vi "2D_rotate.vi"(8 "error in (no error)":errorcluster, 10 "angle":dbl[unit], 11 "input vector":dbl[](array[numeric])) -> (0 "error out":errorcluster, 3 "output vector":dbl[](array[numeric]))   [LabVIEW 2010]
uses:
  <vilib>/Analysis/Matrix/Numeric/Conversions/Array To Matrix - RA2.vi
  <vilib>/Analysis/Matrix/Numeric/Conversions/Array To Matrix - RA.vi
  <vilib>/Analysis/baseanly.llb/Real A x B.vi
  <vilib>/Analysis/Matrix/Numeric/Conversions/Matrix To Array - RM.vi
  <vilib>/Analysis/NI_AALBase.lvlib
  <vilib>/Analysis/Matrix/NI_Matrix.lvlib
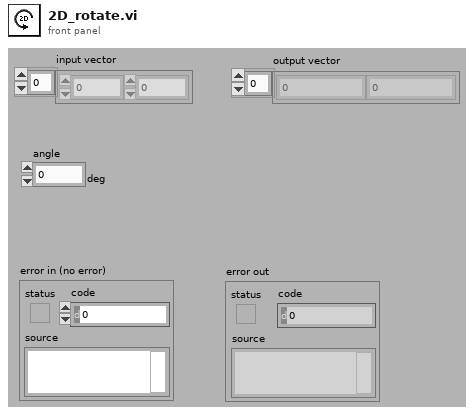
[diagram p1: front panel]
types:
  T1 = typedef "NI_Matrix.lvlib/RealMatrix.ctl" = dbl[][]
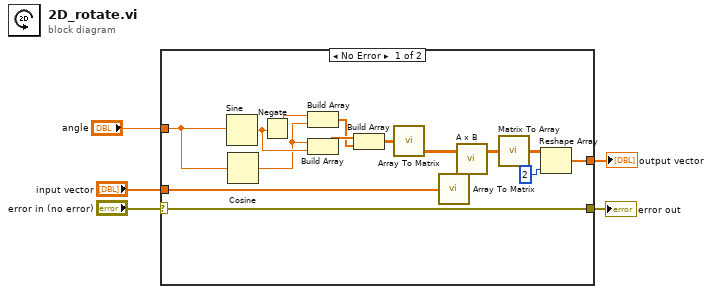
[diagram p0: block diagram]
diagram:
  n1 = case shown="No Error" "error in (no error)" {
    selector: "error in (no error)" -> [w20 w22]
    tunnel: [w20 w22] -> w4
    tunnel: [w8 w21] -> w2
    tunnel: "input vector" -> [w13 w21]
    tunnel: "angle" -> [w19 _]
    frame No Error {
      n2 = Sine(x=w19) -> (sin(x)=w18:dbl)
      n3 = Cosine(x=w19) -> (cos(x)=w16:dbl)
      n4 = Negate(x=w18) -> (-x=w17:dbl)
      n5 = Build Array(w17, w16) -> (w6:dbl[])
      n6 = Build Array(w16, w18) -> (w7:dbl[])
      n7 = Build Array(w7, w6) -> (w15:dbl[][])
      n8 = call-poly <vilib>:"Array To Matrix.vi"("Real 2D Array"=w15) -> ("Real Matrix"=w14:T1)
      n9 = call-poly <vilib>:"Array To Matrix.vi"("Real 1D Array"=w13) -> ("Real Matrix (Column Vector)"=w12:T1)
      n10 = call-poly <vilib>:"A x B.vi"("B"=w12, "A"=w14) -> ("A x B"=w11:T1)  [unwired: 1 out]
      n11 = call-poly <vilib>:"Matrix To Array.vi"("Real Matrix"=w11) -> ("Real 2D Array"=w10:dbl[][])
      n12 = Reshape Array(w10, 2 ("dimension size")) -> (w8:dbl[])
    }
    frame Error {
    }
  }
  "error out" <- w4
  "output vector" <- w2
